vi "GetPIDDataField.vi"(10 "Telemetry Data":string, 11 "Cluster in":refnum<vi>) -> (3 "Array":string[](array[string]))   [LabVIEW 2016]
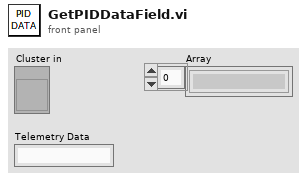
[diagram p1: front panel]
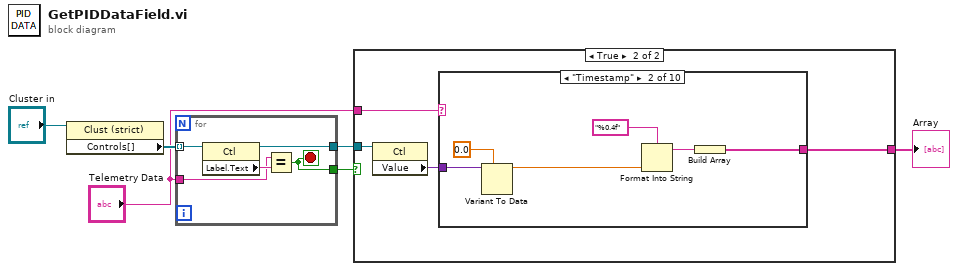
[diagram p0: block diagram]
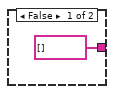
[diagram p2: hidden frame]
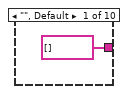
[diagram p3: hidden frame]
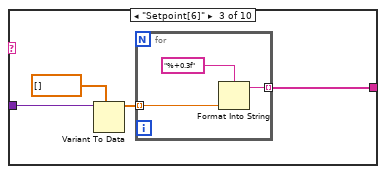
[diagram p4: hidden frame]
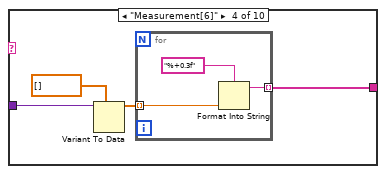
[diagram p5: hidden frame]
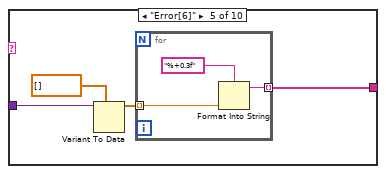
[diagram p6: hidden frame]
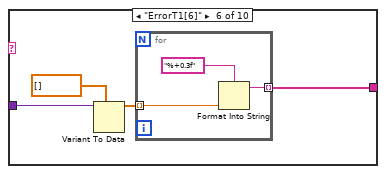
[diagram p7: hidden frame]
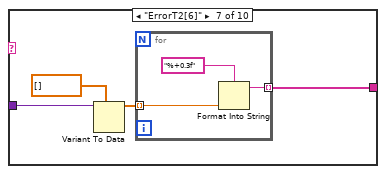
[diagram p8: hidden frame]
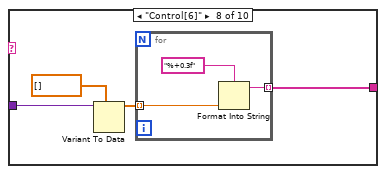
[diagram p9: hidden frame]
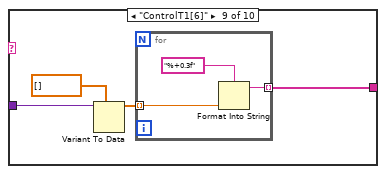
[diagram p10: hidden frame]
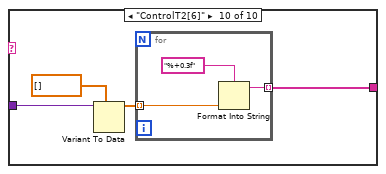
[diagram p11: hidden frame]
diagram:
  n1 = property on="Property Node" class="Clust (strict)"(reference="Cluster in") -> ("Controls[]"=w6:refnum<vi>[])  [unwired: 1 in, 2 out]
  n2 = for {
    tunnel: w6 -> [w11] mode=indexing
    tunnel: [w10] -> w1
    tunnel: "Telemetry Data" -> [w8]
    tunnel: [w7] -> w2
    stop <- w7 stop-if-true
    n3 = property on="Property Node" class="Ctl"(reference=w11) -> (reference out=w10:refnum<vi>, "Label.Text"=w9:string)  [unwired: 1 in, 1 out]
    n4 = Equal?(x=w8, y=w9) -> (x = y?=w7:bool)
  }
  n5 = case shown="True" w2 {
    tunnel: "Telemetry Data" -> [_ w16]
    tunnel: w1 -> [_ w15]
    tunnel: [string[] [] w13] -> w4
    frame False {
    }
    frame True {
      n6 = property on="Property Node" class="Ctl"(reference=w15) -> ("Value"=w14:variant)  [unwired: 1 in, 2 out]
      n7 = case shown="\"Timestamp\"" w16 {
        tunnel: [string[] [] w21 w24 w31 w38 w45 w52 w59 w66 w73] -> w13
        tunnel: w14 -> [_ w19 w27 w34 w41 w48 w55 w62 w69 w76]
        frame "", Default {
        }
        frame "Timestamp" {
          n8 = Variant To Data(type=0.0, Variant=w19) -> (data=w20:dbl)  [unwired: 1 in, 1 out]
          n9 = Format Into String(format string="%0.4f", w20) -> (resulting string=w22:string)  [unwired: 2 in, 1 out]
          n10 = Build Array(w22) -> (w21:string[])
        }
        frame "Setpoint[6]" {
          n11 = Variant To Data(type=sgl[] [], Variant=w27) -> (data=w25:sgl[])  [unwired: 1 in, 1 out]
          n12 = for {
            tunnel: w25 -> [w29] mode=indexing
            tunnel: [w28] -> w24 mode=indexing
            n13 = Format Into String(format string="%+0.3f", w29) -> (resulting string=w28:string)  [unwired: 2 in, 1 out]
          }
        }
        frame "Measurement[6]" {
          n14 = Variant To Data(type=sgl[] [], Variant=w34) -> (data=w32:sgl[])  [unwired: 1 in, 1 out]
          n15 = for {
            tunnel: w32 -> [w36] mode=indexing
            tunnel: [w35] -> w31 mode=indexing
            n16 = Format Into String(format string="%+0.3f", w36) -> (resulting string=w35:string)  [unwired: 2 in, 1 out]
          }
        }
        frame "Error[6]" {
          n17 = Variant To Data(type=sgl[] [], Variant=w41) -> (data=w39:sgl[])  [unwired: 1 in, 1 out]
          n18 = for {
            tunnel: w39 -> [w43] mode=indexing
            tunnel: [w42] -> w38 mode=indexing
            n19 = Format Into String(format string="%+0.3f", w43) -> (resulting string=w42:string)  [unwired: 2 in, 1 out]
          }
        }
        frame "ErrorT1[6]" {
          n20 = Variant To Data(type=sgl[] [], Variant=w48) -> (data=w46:sgl[])  [unwired: 1 in, 1 out]
          n21 = for {
            tunnel: w46 -> [w50] mode=indexing
            tunnel: [w49] -> w45 mode=indexing
            n22 = Format Into String(format string="%+0.3f", w50) -> (resulting string=w49:string)  [unwired: 2 in, 1 out]
          }
        }
        frame "ErrorT2[6]" {
          n23 = Variant To Data(type=sgl[] [], Variant=w55) -> (data=w53:sgl[])  [unwired: 1 in, 1 out]
          n24 = for {
            tunnel: w53 -> [w57] mode=indexing
            tunnel: [w56] -> w52 mode=indexing
            n25 = Format Into String(format string="%+0.3f", w57) -> (resulting string=w56:string)  [unwired: 2 in, 1 out]
          }
        }
        frame "Control[6]" {
          n26 = Variant To Data(type=sgl[] [], Variant=w62) -> (data=w60:sgl[])  [unwired: 1 in, 1 out]
          n27 = for {
            tunnel: w60 -> [w64] mode=indexing
            tunnel: [w63] -> w59 mode=indexing
            n28 = Format Into String(format string="%+0.3f", w64) -> (resulting string=w63:string)  [unwired: 2 in, 1 out]
          }
        }
        frame "ControlT1[6]" {
          n29 = Variant To Data(type=sgl[] [], Variant=w69) -> (data=w67:sgl[])  [unwired: 1 in, 1 out]
          n30 = for {
            tunnel: w67 -> [w71] mode=indexing
            tunnel: [w70] -> w66 mode=indexing
            n31 = Format Into String(format string="%+0.3f", w71) -> (resulting string=w70:string)  [unwired: 2 in, 1 out]
          }
        }
        frame "ControlT2[6]" {
          n32 = Variant To Data(type=sgl[] [], Variant=w76) -> (data=w74:sgl[])  [unwired: 1 in, 1 out]
          n33 = for {
            tunnel: w74 -> [w78] mode=indexing
            tunnel: [w77] -> w73 mode=indexing
            n34 = Format Into String(format string="%+0.3f", w78) -> (resulting string=w77:string)  [unwired: 2 in, 1 out]
          }
        }
      }
    }
  }
  "Array" <- w4
